vi "OPEN Rev-01.vi"(10 "Input Data":dbl[](array[numeric]), 11 "Mean In":dbl=1600.0) -> (3 "OPEN":bool)   [LabVIEW 2012]
uses:
  <vilib>/gmath/NI_Gmath.lvlib
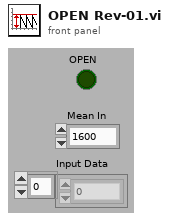
[diagram p1: front panel]
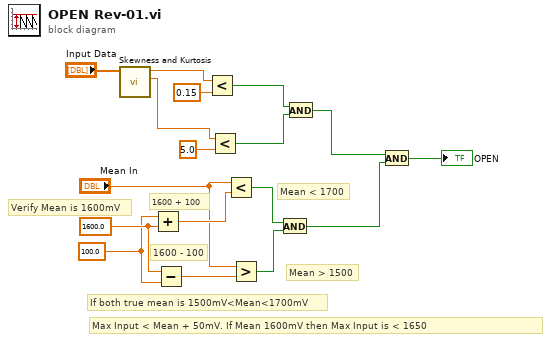
[diagram p0: block diagram]
diagram:
  w15 = 1600.0
  w10 = 100.0
  # "Mean < 1700"
  # "Mean > 1500"
  # "1600 + 100"
  # "1600 - 100"
  # "Max Input < Mean + 50mV. If Mean 1600mV then Max Input is < 1650"
  # "If both true mean is 1500mV<Mean<1700mV"
  # "Verify Mean is 1600mV"
  n1 = call <vilib>:"Skewness and Kurtosis.vi"("X"="Input Data") -> ("kurtosis"=w4:dbl, "skewness"=w5:dbl)  [unwired: 8 in, 1 out]
  n2 = Add(x=w10, y=w15) -> (x+y=w17:dbl)
  n3 = Subtract(x=w15, y=w10) -> (x-y=w16:dbl)
  n4 = Less?(x=w5, y=0.15) -> (x < y?=w3:bool)
  n5 = Less?(x=w4, y=5.0) -> (x < y?=w2:bool)
  n6 = Less?(x="Mean In", y=w17) -> (x < y?=w14:bool)
  n7 = Greater?(x="Mean In", y=w16) -> (0:w13:bool)
  n8 = And(x=w14, y=w13) -> (x .and. y?=w12:bool)
  n9 = And(x=w3, y=w2) -> (x .and. y?=w9:bool)
  n10 = And(x=w9, y=w12) -> (x .and. y?=→"OPEN":bool)
